vi "Translator.MainGui.vi"(6 "~Do not save font? (F)":bool, 7 "~init (F)":bool, 8 "~error in":errorcluster, 10 "~Language in use":string="English", 11 "~Translation folder":path=path "D:/PL_0125_Sapphire_Automation_branches/SOFTWARE_v1.1-Translation/settings") -> (0 "~error out":errorcluster, 1 "~restart?":bool, 2 "~font name":string, 4 "~flag small":picture)   [LabVIEW 2016]
uses:
  <vilib>/Utility/miscctls.llb/LVBoundsTypeDef.ctl
  Translator.Global.vi
panel:
  out "~progressbar2":i32(slide) scale=-1.1..7.0
  out "~progressbar1":i32(slide) scale=-1.1..-1.0
  out "Message":string
  out "~flag":picture
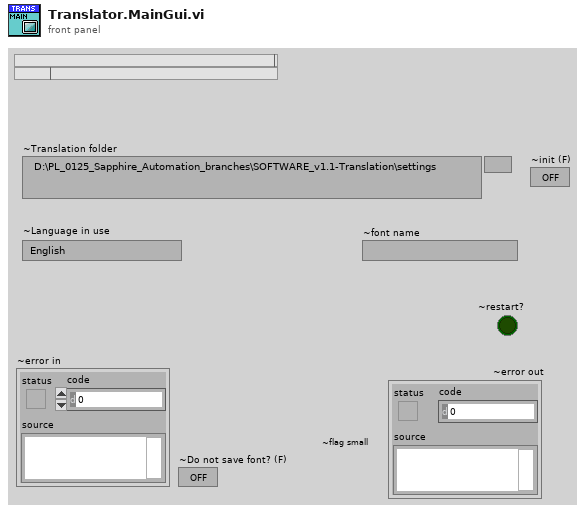
[diagram p1: front panel]
types:
  T1 = typedef "LVBoundsTypeDef.ctl" = cluster{"Width":u32, "Height":u32}
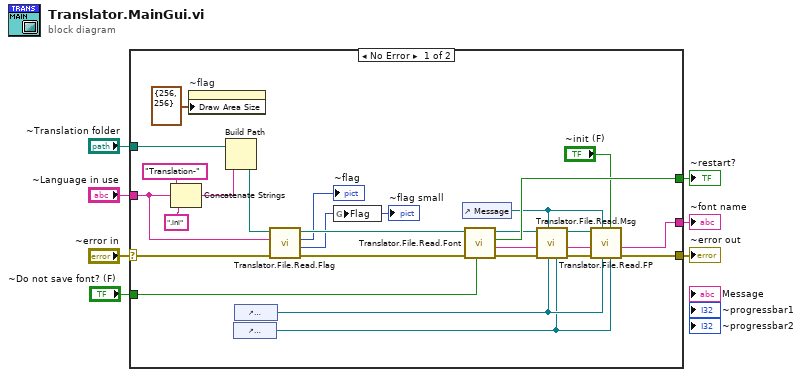
[diagram p0: block diagram]
diagram:
  n1 = case shown="No Error" "~error in" {
    selector: "~error in" -> [w21 w29]
    tunnel: "~Translation folder" -> [w17 _]
    tunnel: [w15 w29] -> w4
    tunnel: "~Language in use" -> [w20 _]
    tunnel: [w16 _] -> w3
    tunnel: [w23 _] -> w2
    tunnel: "~Do not save font? (F)" -> [w18 _]
    frame No Error {
      n2 = Concatenate Strings("Translation-" ("string"), w20, ".ini" ("string")) -> (w26:string)
      n3 = property on="~flag" class="Pict"("Draw Area Size"=T1 {"Width"=256, "Height"=256}) -> ()  [unwired: 2 in, 2 out]
      n4 = Build Path(base path=w17, name or relative path=w26) -> (appended path=w22:path)
      n5 = control-ref of="~progressbar2"() -> (w24:refnum<vi>)
      n6 = control-ref of="~progressbar1"() -> (w25:refnum<vi>)
      n7 = call "Translator.File.Read.Flag.vi"("error in"=w21, "Language in use"=w20, "Translation file"=w22) -> ("error out"=w10:errorcluster, "~flag small"=w8:picture, "~flag"=→"~flag":picture)  [unwired: 6 in]
      "~flag small" <- w8
      n8 = global write "Translator.Global.vi" "Flag"(w8) -> ()
      n9 = control-ref of="Message"() -> (w14:refnum<vi>)
      n10 = call "Translator.File.Read.Font.vi"("Do not save font? (F)"=w18, "error in"=w10, "Translation file"=w22) -> ("error out"=w13:errorcluster, "font name"=w16:string, "restart required?"=w23:bool)  [unwired: 6 in]
      n11 = call "Translator.File.Read.Msg.vi"("progressbar2"=w24, "progressbar1"=w25, "Message"=w14, "error in"=w13, "Translation folder"=w22) -> ("error out"=w12:errorcluster)  [unwired: 6 in]
      n12 = call "Translator.File.Read.FP.vi"("progressbar2"=w24, "init"="~init (F)", "progressbar1"=w25, "Message"=w14, "error in"=w12, "font name"=w16, "Translation file"=w22) -> ("error out"=w15:errorcluster)  [unwired: 4 in]
    }
    frame Error {
    }
  }
  "~error out" <- w4
  "~font name" <- w3
  "~restart?" <- w2
